vi "TestNotifierBehavior.vi"() -> ()   [LabVIEW 2013]
panel:
  out "Grab 4":T1
  out "Grab 3":T1
  out "Grab 2":T1
  out "Grab 1":T1
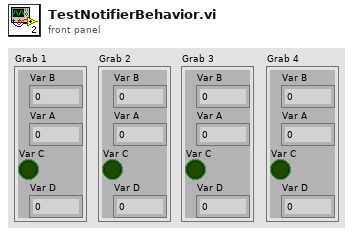
[diagram p1: front panel]
types:
  T1 = cluster{"Var B":dbl, "Var A":dbl, "Var C":bool, "Var D":i32}
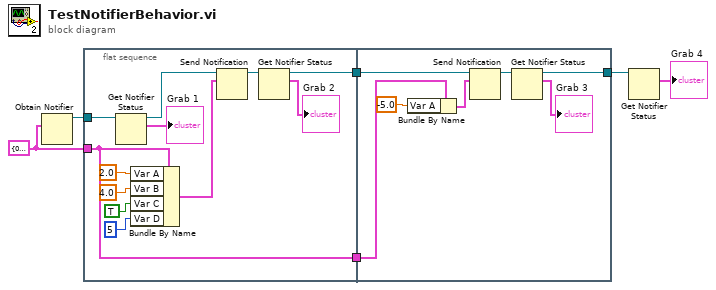
[diagram p0: block diagram]
diagram:
  w5 = T1 {"Var B"=0.0, "Var A"=0.0, "Var C"=FALSE, "Var D"=0}
  n1 = Obtain Notifier(notification data type=w5) -> (notifier out=w6:refnum<notifier>)  [unwired: 3 in, 2 out]
  n2 = flat-sequence {
    tunnel: w6 -> [w18]
    tunnel: w5 -> [w7]
    tunnel: [w8] -> w4
    tunnel: [w7] -> w3
    tunnel: w4 -> [w25]
    tunnel: w3 -> [w24]
    tunnel: [w19] -> w2
    frame #0 {
      n3 = Get Notifier Status(notifier=w18) -> (notifier out=w16:refnum<notifier>, current notification=→"Grab 1":T1)  [unwired: 1 in, 3 out]
      n4 = Bundle By Name(cluster=w7, "Var A"=2.0, "Var B"=4.0, "Var C"=TRUE, "Var D"=5) -> (w9:T1)
      n5 = Send Notification(notification=w9, notifier=w16) -> (notifier out=w14:refnum<notifier>)  [unwired: 1 in, 1 out]
      n6 = Get Notifier Status(notifier=w14) -> (notifier out=w8:refnum<notifier>, current notification=→"Grab 2":T1)  [unwired: 1 in, 3 out]
    }
    frame #1 {
      n7 = Bundle By Name(cluster=w24, "Var A"=-5.0) -> (w22:T1)
      n8 = Send Notification(notification=w22, notifier=w25) -> (notifier out=w21:refnum<notifier>)  [unwired: 1 in, 1 out]
      n9 = Get Notifier Status(notifier=w21) -> (notifier out=w19:refnum<notifier>, current notification=→"Grab 3":T1)  [unwired: 1 in, 3 out]
    }
  }
  n10 = Get Notifier Status(notifier=w2) -> (current notification=→"Grab 4":T1)  [unwired: 1 in, 4 out]
